vi "Enum - DropPolicy and FilterMode.vi"(8 "error in (no error)":errorcluster) -> (0 "error out":errorcluster)   [LabVIEW 2026, in "Tests.lvlib"]
doc: "Unit test (Caraya) for the DropPolicy and FilterMode name<->enum mappers.\nRound-trips each member name through FromString then String and asserts the original name comes back, guarding the I32-vs-U16 Type Cast bug that made FromString return the ordinal-0 member. Also asserts an unknown name faults with its specific code.\nPure test: no actors, no file I/O.\n\nImplements LMBR-T-060 -> SRS-050a; LMBR-T-025 (DropPolicy, FilterMode) -> SRS-048. Assert-level IDs: Test-ID-Assert-Checklist.md."
uses:
  Tests.lvlib
  <vilib>/addons/_JKI Toolkits/Caraya/classes/Assert/Assert Equal Value_Variant.vi
  <vilib>/addons/_JKI Toolkits/Caraya/classes/Assert/Assert Not Error.vi
  <vilib>/addons/_JKI Toolkits/Caraya/classes/Assert/Assert Error.vi
  <vilib>/addons/_JKI Toolkits/Caraya/classes/Assert/Assert True.vi
  <vilib>/addons/_JKI Toolkits/Caraya/classes/Test/Test.lvclass
  src/Lumberjack.lvlib
  <vilib>/addons/_JKI Toolkits/Caraya/classes/Assert/Assert.lvclass
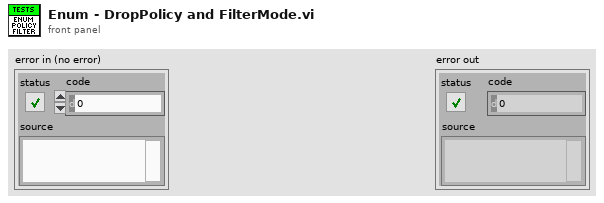
[diagram p1: front panel]
types:
  T1 = typedef "Lumberjack.lvlib/DropPolicy.ctl" = enum16{"DropOldest", "DropNewest", "LevelAware"}
  T2 = typedef "Lumberjack.lvlib/FilterMode.ctl" = enum16{"Mirror", "Routed"}
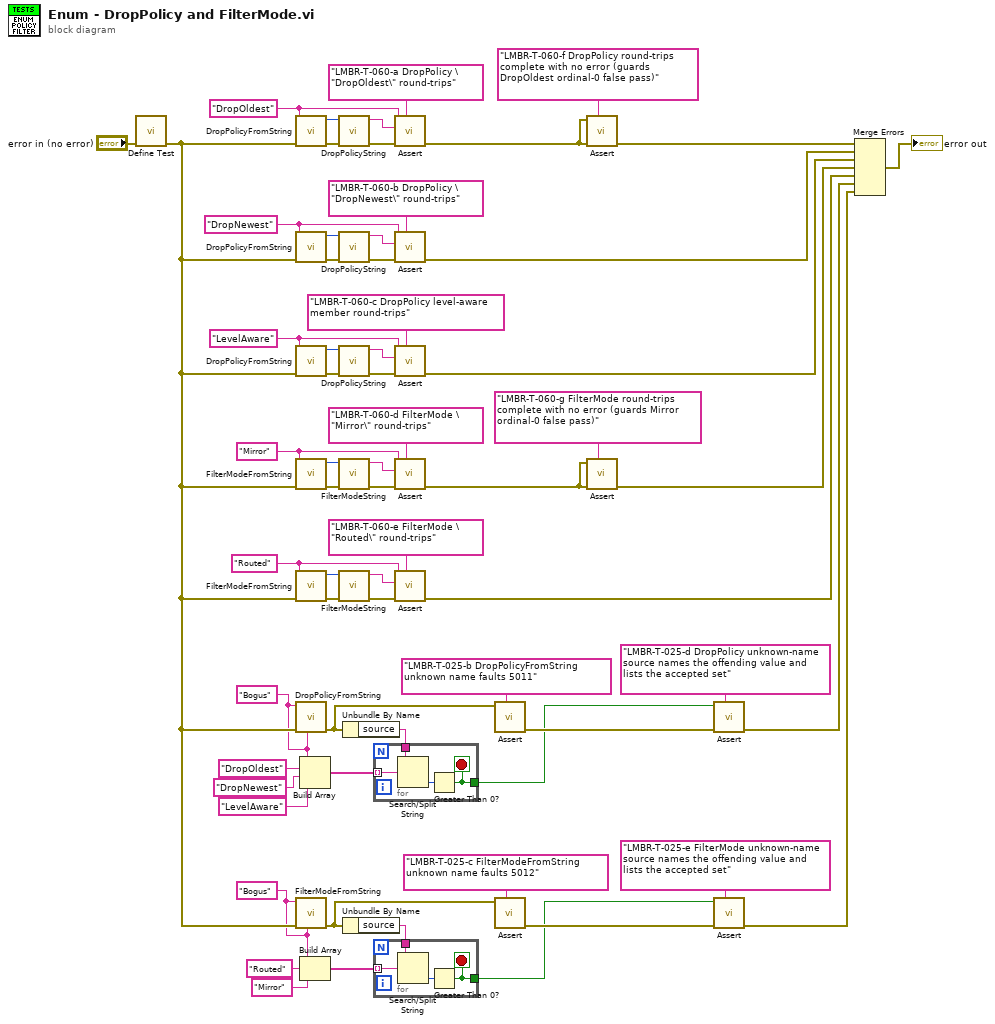
[diagram p0: block diagram]
diagram:
  w16 = "Bogus" ("DropPolicyString")
  w15 = "Bogus" ("FilterModeString")
  w33 = "Routed" ("FilterModeString")
  w40 = "LevelAware" ("DropPolicyString")
  w47 = "DropNewest" ("DropPolicyString")
  w54 = "Mirror" ("FilterModeString")
  w59 = "DropOldest" ("DropPolicyString")
  n1 = call <vilib>:"Define Test.vi"("error in (no error)"="error in (no error)") -> ("error out"=w22:errorcluster)  [unwired: 9 in, 1 out]
  n2 = call "DropPolicyFromString.vi"("error in (no error)"=w22, "DropPolicyString"=w59) -> ("error out"=w62:errorcluster, "DropPolicy"=w63:T1)  [unwired: 8 in]
  n3 = call "DropPolicyFromString.vi"("error in (no error)"=w22, "DropPolicyString"=w47) -> ("error out"=w50:errorcluster, "DropPolicy"=w51:T1)  [unwired: 8 in]
  n4 = call "DropPolicyFromString.vi"("error in (no error)"=w22, "DropPolicyString"=w40) -> ("error out"=w43:errorcluster, "DropPolicy"=w44:T1)  [unwired: 8 in]
  n5 = call "FilterModeFromString.vi"("error in (no error)"=w22, "FilterModeString"=w54) -> ("error out"=w58:errorcluster, "FilterMode"=w56:T2)  [unwired: 8 in]
  n6 = call "FilterModeFromString.vi"("error in (no error)"=w22, "FilterModeString"=w33) -> ("error out"=w37:errorcluster, "FilterMode"=w35:T2)  [unwired: 8 in]
  n7 = call "DropPolicyFromString.vi"("Context"=w16, "error in (no error)"=w22, "DropPolicyString"=w16) -> ("error out"=w14:errorcluster)  [unwired: 7 in, 1 out]
  n8 = call "FilterModeFromString.vi"("Context"=w15, "error in (no error)"=w22, "FilterModeString"=w15) -> ("error out"=w13:errorcluster)  [unwired: 7 in, 1 out]
  n9 = Build Array(w16, "DropOldest", "DropNewest", "LevelAware") -> (w12:string[])
  n10 = Build Array(w15, "Routed", "Mirror") -> (w9:string[])
  n11 = call "DropPolicyString.vi"("error in (no error)"=w62, "DropPolicy"=w63) -> ("error out"=w61:errorcluster, "DropPolicyString"=w60:string)  [unwired: 8 in]
  n12 = call "DropPolicyString.vi"("error in (no error)"=w50, "DropPolicy"=w51) -> ("error out"=w49:errorcluster, "DropPolicyString"=w48:string)  [unwired: 8 in]
  n13 = call "DropPolicyString.vi"("error in (no error)"=w43, "DropPolicy"=w44) -> ("error out"=w42:errorcluster, "DropPolicyString"=w41:string)  [unwired: 8 in]
  n14 = call "FilterModeString.vi"("error in (no error)"=w58, "FilterMode"=w56) -> ("error out"=w57:errorcluster, "FilterModeString"=w55:string)  [unwired: 8 in]
  n15 = call "FilterModeString.vi"("error in (no error)"=w37, "FilterMode"=w35) -> ("error out"=w36:errorcluster, "FilterModeString"=w34:string)  [unwired: 8 in]
  n16 = Unbundle By Name(w14) -> ("source"=w11:string)
  n17 = Unbundle By Name(w13) -> ("source"=w10:string)
  n18 = for {
    tunnel: w12 -> [w68] mode=indexing
    tunnel: w11 -> [w69]
    tunnel: [w66] -> w7
    stop <- w66 stop-if-true
    n19 = Search/Split String(string=w69, search string/char (-)=w68) -> (offset of match=w67:i32)  [unwired: 1 in, 2 out]
    n20 = Greater Than 0?(x=w67) -> (x > 0?=w66:bool)
  }
  n21 = for {
    tunnel: w9 -> [w72] mode=indexing
    tunnel: w10 -> [w73]
    tunnel: [w70] -> w3
    stop <- w70 stop-if-true
    n22 = Search/Split String(string=w73, search string/char (-)=w72) -> (offset of match=w71:i32)  [unwired: 1 in, 2 out]
    n23 = Greater Than 0?(x=w71) -> (x > 0?=w70:bool)
  }
  n24 = call-poly <vilib>:"Assert.vi"("Label"="LMBR-T-060-a DropPolicy \"DropOldest\" round-trips", "error in (no error)"=w61, "Actual"=w60, "Expected"=w59) -> ("error out"=w29:errorcluster)  [unwired: 6 in, 1 out]
  n25 = call-poly <vilib>:"Assert.vi"("Label"="LMBR-T-060-b DropPolicy \"DropNewest\" round-trips", "error in (no error)"=w49, "Actual"=w48, "Expected"=w47) -> ("error out"=w45:errorcluster)  [unwired: 6 in, 1 out]
  n26 = call-poly <vilib>:"Assert.vi"("Label"="LMBR-T-060-c DropPolicy level-aware member round-trips", "error in (no error)"=w42, "Actual"=w41, "Expected"=w40) -> ("error out"=w38:errorcluster)  [unwired: 6 in, 1 out]
  n27 = call-poly <vilib>:"Assert.vi"("Label"="LMBR-T-060-d FilterMode \"Mirror\" round-trips", "error in (no error)"=w57, "Actual"=w55, "Expected"=w54) -> ("error out"=w28:errorcluster)  [unwired: 6 in, 1 out]
  n28 = call-poly <vilib>:"Assert.vi"("Label"="LMBR-T-060-e FilterMode \"Routed\" round-trips", "error in (no error)"=w36, "Actual"=w34, "Expected"=w33) -> ("error out"=w31:errorcluster)  [unwired: 6 in, 1 out]
  n29 = call-poly <vilib>:"Assert.vi"("Label"="LMBR-T-025-b DropPolicyFromString unknown name faults 5011", "Error?"=w14) -> ("error out"=w8:errorcluster)  [unwired: 8 in, 1 out]
  n30 = call-poly <vilib>:"Assert.vi"("Label"="LMBR-T-025-c FilterModeFromString unknown name faults 5012", "Error?"=w13) -> ("error out"=w4:errorcluster)  [unwired: 8 in, 1 out]
  n31 = call-poly <vilib>:"Assert.vi"("Label"="LMBR-T-060-f DropPolicy round-trips complete with no error (guards DropOldest ordinal-0 false pass)", "error in (no error)"=w29, "Not Error?"=w29) -> ("error out"=w30:errorcluster)  [unwired: 7 in, 1 out]
  n32 = call-poly <vilib>:"Assert.vi"("Label"="LMBR-T-060-g FilterMode round-trips complete with no error (guards Mirror ordinal-0 false pass)", "error in (no error)"=w28, "Not Error?"=w28) -> ("error out"=w27:errorcluster)  [unwired: 7 in, 1 out]
  n33 = call-poly <vilib>:"Assert.vi"("Label"="LMBR-T-025-d DropPolicy unknown-name source names the offending value and lists the accepted set", "error in (no error)"=w8, "True?"=w7) -> ("error out"=w2:errorcluster)  [unwired: 7 in, 1 out]
  n34 = call-poly <vilib>:"Assert.vi"("Label"="LMBR-T-025-e FilterMode unknown-name source names the offending value and lists the accepted set", "error in (no error)"=w4, "True?"=w3) -> ("error out"=w1:errorcluster)  [unwired: 7 in, 1 out]
  n35 = Merge Errors(w30, w45, w38, w27, w31, w2, w1) -> (→"error out":errorcluster)
